vi "Set settings chain.vi"(8 "error in (no error)":errorcluster, 9 "class name":string[](array[string]), 10 "settings":variant[](array[variant]), 11 "ExampleClassB in":refnum<class "ExampleClassB.lvclass">) -> (0 "error out":errorcluster, 3 "ExampleClassB out":refnum<class "ExampleClassB.lvclass">)   [LabVIEW 2012, in "ExampleClassB.lvclass"]
uses:
  ExampleClassB.lvclass
  ExampleClassB.lvclass/ExampleClassB.ctl
  <vilib>/Distrio/Murmex/Murmex/Murmex.lvclass
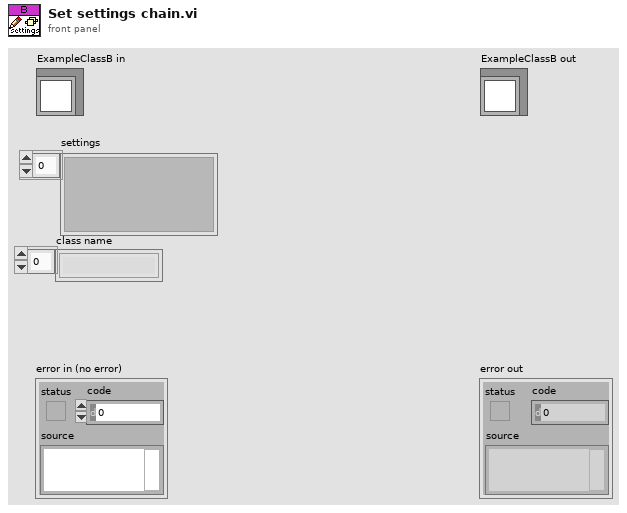
[diagram p1: front panel]
types:
  T1 = typedef "ExampleClassB.lvclass/Settings cluster.ctl" = cluster{"expected samples":i32}
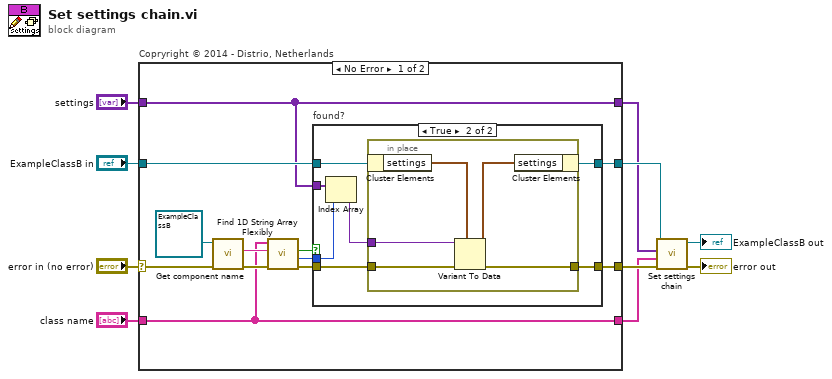
[diagram p0: block diagram]
diagram:
  n1 = case "Copryright © 2014 - Distrio, Netherlands" shown="No Error" "error in (no error)" {
    selector: "error in (no error)" -> [w22 w40]
    tunnel: [w20 w40] -> w8
    tunnel: [w21 w39] -> w6
    tunnel: "ExampleClassB in" -> [w14 w39]
    tunnel: "class name" -> [w11 w37]
    tunnel: "settings" -> [w12 w38]
    tunnel: [w12 w38] -> w3
    tunnel: [w11 w37] -> w2
    frame No Error {
      n2 = call <vilib>:"Get component name.vi"("error in (no error)"=w22, "Murmex in"=refnum<class "ExampleClassB.lvclass"> refnum ("ExampleClassB in")) -> ("error out"=w19:errorcluster, "component name"=w17:string)  [unwired: 7 in, 1 out]
      n3 = call <vilib>:"Find 1D String Array Flexibly.vi"("error in (no error)"=w19, "element"=w17, "array"=w11) -> ("error out"=w18:errorcluster, "index of element"=w16:i32, "found?"=w15:bool)  [unwired: 6 in]
      n4 = case "found?" shown="True" w15 {
        tunnel: w12 -> [_ w31]
        tunnel: w14 -> [w24 w29]
        tunnel: [w24 w28] -> w21
        tunnel: [w23 w27] -> w20
        tunnel: w18 -> [w23 w26]
        tunnel: w16 -> [_ w25]
        frame False {
        }
        frame True {
          n5 = Index Array(array=w31, index=w25) -> (element=w30:variant)
          n6 = in-place {
            in-place-border: w30 -> [w36]
            in-place-border: w26 -> [w34]
            in-place-border: [w32] -> w27
            n7 = in-place-cluster #1(w29) -> ("settings"=w35:T1)
            n8 = Variant To Data(error in=w34, type=w35, Variant=w36) -> (data=w33:T1, error out=w32:errorcluster)
            n9 = in-place-cluster #1("settings"=w33) -> (w28:refnum<class "ExampleClassB.lvclass">)
          }
        }
      }
    }
    frame Error {
    }
  }
  n10 = call-parent "Set settings chain.vi"("error in (no error)"=w8, "class names"=w2, "settings"=w3, "Murmex in"=w6) -> ("error out"=→"error out":errorcluster, "Murmex out"=→"ExampleClassB out":refnum<class "ExampleClassB.lvclass">)  [unwired: 6 in]
